vi "thorlabs_stop_polling.vi"(8 "error in (no error)":errorcluster, 10 "channel":i16, 11 "thorlabs_kinesis in":refnum<class "thorlabs_kinesis.lvclass">) -> (0 "error out":errorcluster, 3 "thorlabs_kinesis out":refnum<class "thorlabs_kinesis.lvclass">)   [LabVIEW 2015, in "thorlabs_kinesis.lvclass"]
uses:
  thorlabs_kinesis.lvclass
  thorlabs_kinesis.lvclass/thorlabs_kinesis.ctl
  thorlabs_drivers/Thorlabs.MotionControl.Benchtop.Piezo.dll
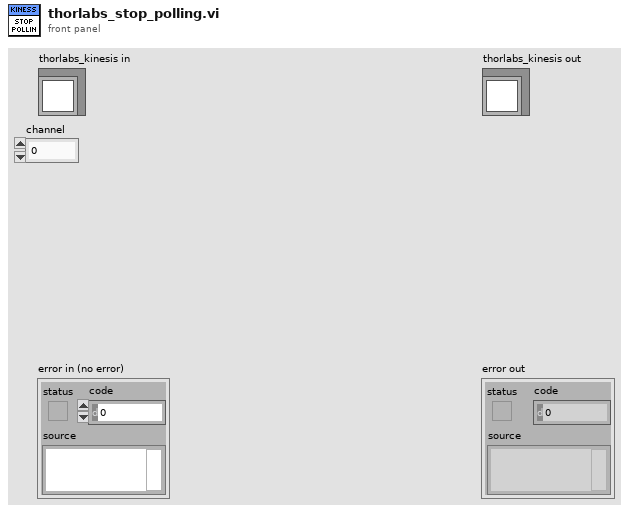
[diagram p1: front panel]
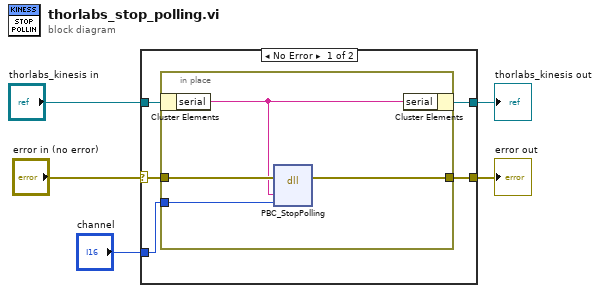
[diagram p0: block diagram]
diagram:
  n1 = case shown="No Error" "error in (no error)" {
    selector: "error in (no error)" -> [w10 w16]
    tunnel: [w6 w16] -> w4
    tunnel: [w7 w15] -> w2
    tunnel: "thorlabs_kinesis in" -> [w8 w15]
    tunnel: "channel" -> [w9 _]
    frame No Error {
      n2 = in-place {
        in-place-border: w10 -> [w14]
        in-place-border: w9 -> [w13]
        in-place-border: [w11] -> w6
        n3 = in-place-cluster #1(w8) -> ("serial"=w12:string)
        n4 = dll-call lib="C:/Users/bspoka/Documents/LabVIEW Data/lview_180307/Stage Class/Thorlabs Kinesis/thorlabs_drivers/Thorlabs.MotionControl.Benchtop.Piezo.dll" fn="PBC_StopPolling" label="PBC_StartPolling"(error in=w14, "serial"=w12, "channel"=w13) -> (error out=w11:errorcluster)  [unwired: 5 in, 1 out]
        n5 = in-place-cluster #1("serial"=w12) -> (w7:refnum<class "thorlabs_kinesis.lvclass">)
      }
    }
    frame Error {
    }
  }
  "error out" <- w4
  "thorlabs_kinesis out" <- w2
